vi "Load Config.vi"(8 "error in (no error)":errorcluster) -> (0 "error out":errorcluster, 3 "Config":T1)   [LabVIEW 2018, in "Config File.lvlib"]
uses:
  Config File.lvlib
  Config Cluster.ctl
  Track Info/Track Info.ctl
  <vilib>/Utility/xml.llb/Read From XML File(string).vi
  Track Info/Track Info.lvlib
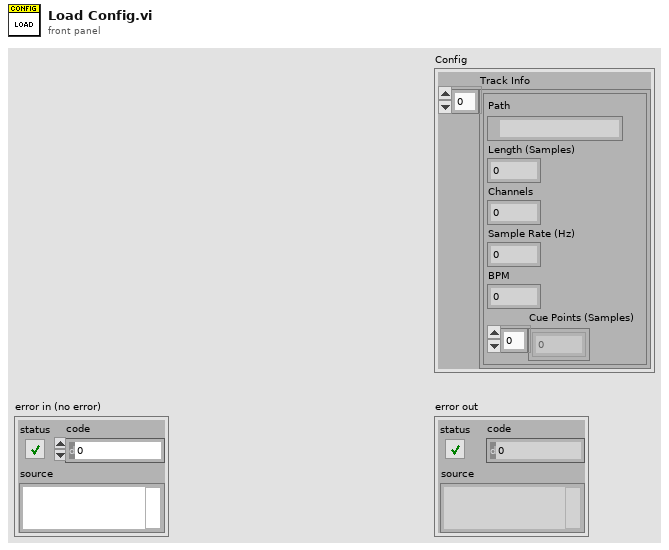
[diagram p1: front panel]
types:
  T1 = typedef "Config File.lvlib/Config Cluster.ctl" = cluster{"Track Info":T2[]}
  T2 = typedef "Track Info.lvlib/Track Info.ctl" = cluster{"Path":path, "Length (Samples)":i32, "Channels":i32, "Sample Rate (Hz)":i32, "BPM":dbl, "Cue Points (Samples)":i32[]}
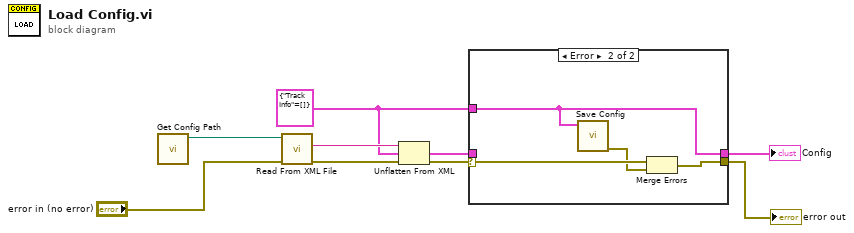
[diagram p0: block diagram]
diagram:
  w5 = T1 {"Track Info"=[]} ("Config")
  n1 = call "Get Config Path.vi"() -> ("Config Path"=w6:path)  [unwired: 11 in]
  n2 = call-poly <vilib>:"Read From XML File.vi"("error in (no error)"="error in (no error)", "XML File Path"=w6) -> ("error out"=w8:errorcluster, "XML Elements"=w9:string)  [unwired: 7 in, 1 out]
  n3 = Unflatten From XML(xml string=w9, type=w5, error in (no error)=w8) -> (value=w7:T1, error out=w2:errorcluster)
  n4 = case shown="Error" w2 {
    selector: w2 -> [w10 w14]
    tunnel: w7 -> [w11 _]
    tunnel: [w11 w15] -> w4
    tunnel: w5 -> [_ w15]
    tunnel: [w10 w12] -> w1
    frame No Error {
    }
    frame Error {
      n5 = call "Save Config.vi"("Config"=w15) -> ("error out"=w13:errorcluster)  [unwired: 10 in]
      n6 = Merge Errors(w14, w13) -> (w12:errorcluster)
    }
  }
  "error out" <- w1
  "Config" <- w4
